vi "AD（V2.0）.vi"() -> (1 "时域谱":dbl[](graph), 2 "幅频谱":dbl[](graph))   [LabVIEW 2016]
uses:
  <vilib>/Analysis/2dsp.llb/Real FFT.vi
  <vilib>/Analysis/NI_AALPro.lvlib
panel:
  out "数值":i32
  # "[220，2000]"
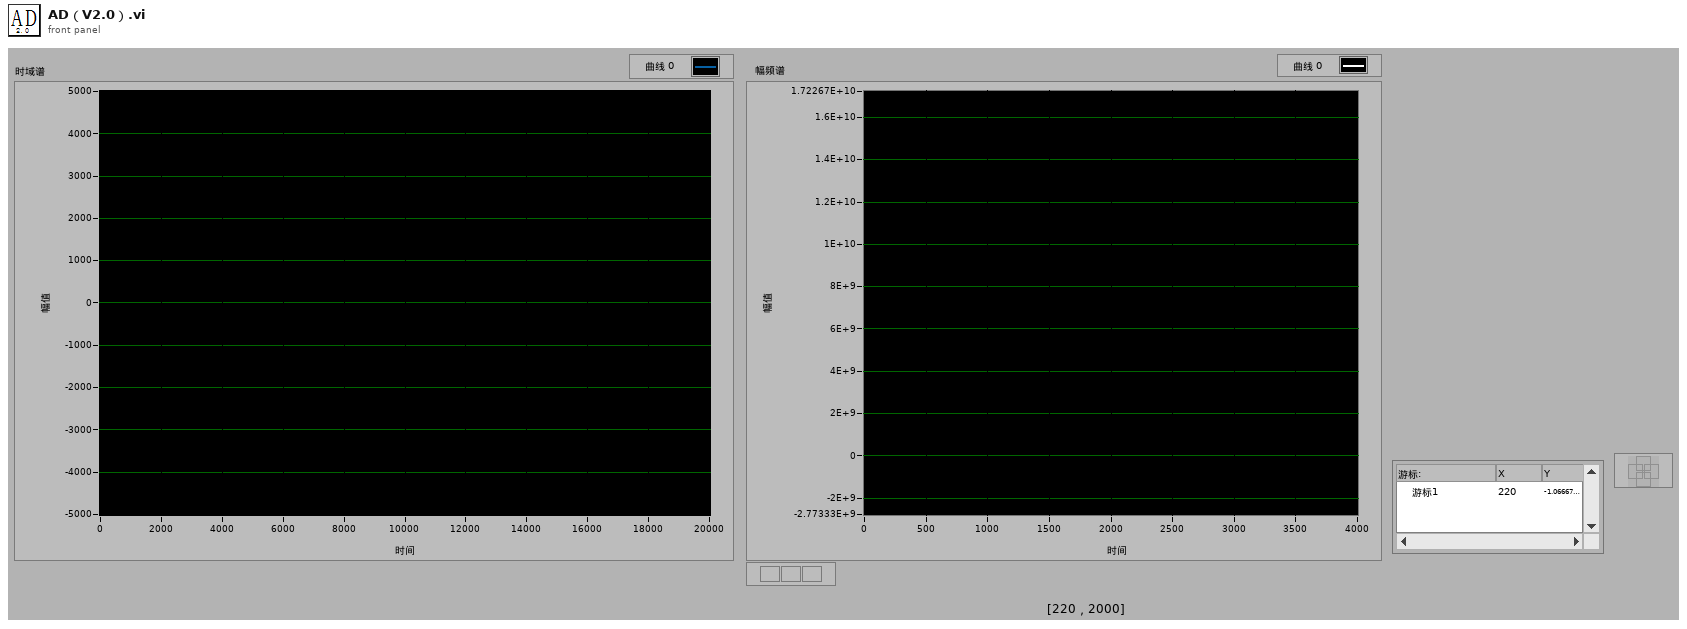
[diagram p1: front panel]
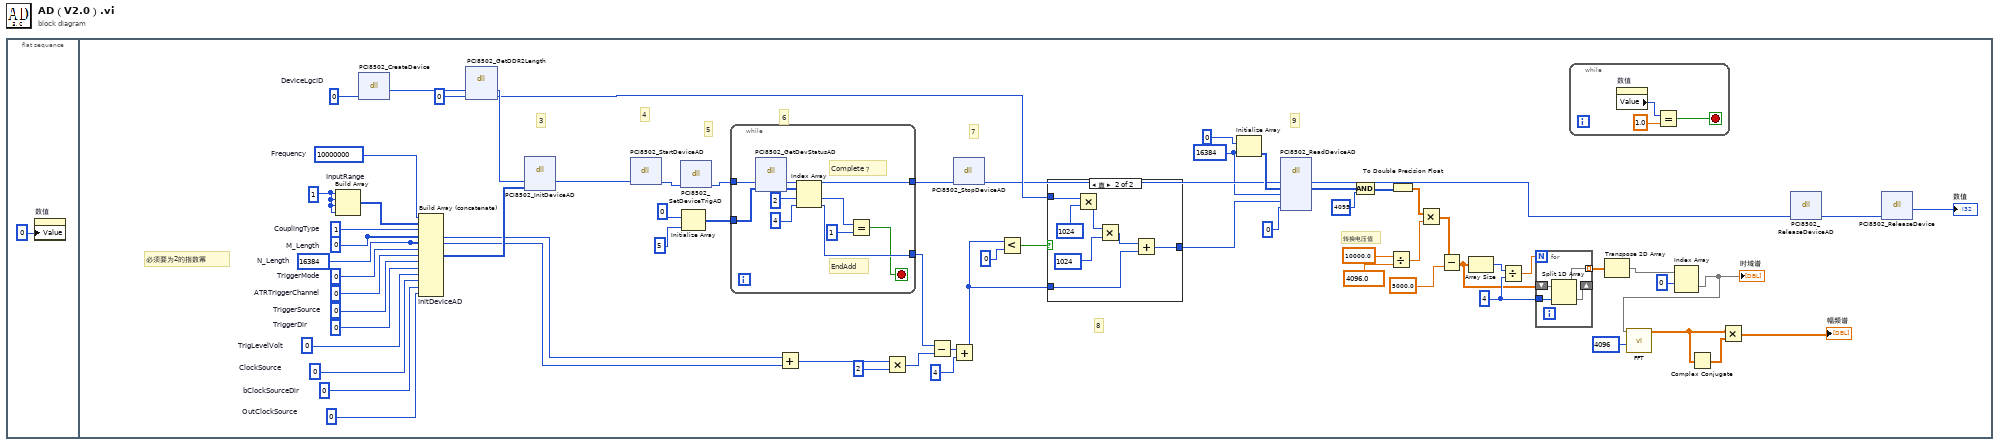
[diagram p0: block diagram]
diagram:
  n1 = flat-sequence {
    frame #0 {
      n2 = property on="数值" class="DigNum (严格)"("Value"=0 ("数值")) -> ()  [unwired: 2 in, 2 out]
    }
    frame #1 {
      w2 = 0  # DeviceLgcID
      w16 = 4
      w18 = 16384 ("dimension size")
      w57 = 0  # OutClockSource
      w58 = 0  # bClockSourceDir
      w60 = 10000000  # Frequency
      w61 = 0  # ClockSource
      w62 = 0  # TrigLevelVolt
      w5 = 1
      w63 = 0  # TriggerDir
      w64 = 0  # TriggerSource
      w65 = 0  # ATRTriggerChannel
      w66 = 0  # TriggerMode
      w49 = 16384  # N_Length
      w50 = 0  # M_Length
      w67 = 1  # CouplingType
      # "9"
      # "8"
      # "7"
      # "6"
      # "5"
      # "4"
      # "转换电压值"
      # "3"
      # "必须要为2的指数幂"
      n3 = Build Array "InputRange"(w5, w5, w5, w5) -> (w4:i32[])
      n4 = dll-call lib="PTH2]abs CUsersH301Desktopart闭环扫描程序采集卡控制INFamd64\nPCI8502_32" fn="PCI8502_CreateDevice" label="CreateDevice"("DeviceLgcID"=w2) -> (w55:i32)  [unwired: 4 in, 2 out]
      n5 = Build Array (concatenate) "InitDeviceAD"(w60, w4, w67, w50, w49, w66, w65, w64, w63, w62, w61, w58, w57) -> (w59:i32[])
      n6 = dll-call lib="PTH2]abs CUsersH301Desktopart闭环扫描程序采集卡控制INFamd64\nPCI8502_32" fn="PCI8502_GetDDR2Length" label="GetDDR2Length"("hDevice"=w55, "pulDDR2Length"=u32 0) -> ("hDevice"=w54:i32, "pulDDR2Length"=w52:u32)  [unwired: 4 in, 2 out]
      n7 = dll-call lib="PTH2]abs CUsersH301Desktopart闭环扫描程序采集卡控制INFamd64\nPCI8502_32" fn="PCI8502_InitDeviceAD" label="InitDeviceAD"("hDevice"=w54, "pADPara"=w59) -> ("hDevice"=w56:i32)  [unwired: 5 in, 2 out]
      n8 = dll-call lib="PTH2]abs CUsersH301Desktopart闭环扫描程序采集卡控制INFamd64\nPCI8502_32" fn="PCI8502_StartDeviceAD" label="StartDeviceAD"("hDevice"=w56) -> ("hDevice"=w47:i32)  [unwired: 4 in, 2 out]
      n9 = dll-call lib="PTH2]abs CUsersH301Desktopart闭环扫描程序采集卡控制INFamd64\nPCI8502_32" fn="PCI8502_SetDeviceTrigAD" label="SetDeviceTrigAD"("hDevice"=w47) -> ("hDevice"=w25:i32)  [unwired: 4 in, 2 out]
      n10 = Initialize Array(0, 5) -> (w22:i32[])
      n11 = while {
        tunnel: [w79] -> w21
        tunnel: w25 -> [w78]
        tunnel: w22 -> [w77]
        tunnel: [w76] -> w19
        stop <- w75 stop-if-true
        # "EndAdd"
        # "Complete？"
        n12 = dll-call lib="PTH2]abs CUsersH301Desktopart闭环扫描程序采集卡控制INFamd64\nPCI8502_32" fn="PCI8502_GetDevStatusAD" label="GetDevStatusAD"("hDevice"=w78, "pADStatus"=w77) -> ("hDevice"=w76:i32, "pADStatus"=w81:i32[])  [unwired: 4 in, 2 out]
        n13 = Index Array(array=w81, index #1=2, index #2=4) -> (element #1=w83:i32, element #2=w79:i32)
        n14 = Equal?(x=w83, y=1) -> (x = y?=w75:bool)
      }
      n15 = Add(x=w50, y=w49) -> (x+y=w20:i32)
      n16 = Multiply(x=w20, y=u32 2) -> (x*y=w33:u32)
      n17 = Subtract(x=w21, y=w33) -> (x-y=w35:u32)
      n18 = Add(x=w35, y=u32 4) -> (x+y=w30:u32)
      n19 = dll-call lib="PTH2]abs CUsersH301Desktopart闭环扫描程序采集卡控制INFamd64\nPCI8502_32" fn="PCI8502_StopDeviceAD" label="StopDeviceAD"("hDevice"=w19) -> ("hDevice"=w36:i32)  [unwired: 4 in, 2 out]
      n20 = Less?(x=w30, y=u32 0) -> (x < y?=w26:bool)
      n21 = case shown="真" w26 {
        tunnel: w30 -> [w85 w88]
        tunnel: [w85 w87] -> w31
        tunnel: w52 -> [_ w86]
        frame False {
        }
        frame True {
          n22 = Multiply(x=w86, y=u32 1024) -> (x*y=w91:u32)
          n23 = Multiply(x=w91, y=u32 1024) -> (x*y=w89:u32)
          n24 = Add(x=w89, y=w88) -> (x+y=w87:u32)
        }
      }
      n25 = Initialize Array(0, w18) -> (w37:i32[])
      n26 = dll-call lib="PTH2]abs CUsersH301Desktopart闭环扫描程序采集卡控制INFamd64\nPCI8502_32" fn="PCI8502_ReadDeviceAD" label="ReadDeviceAD"("hDevice"=w36, "ADBuffer"=w37, "nReadSizeWords"=w18, "ulStartAddr"=w31, "nRetSizeWords"=0) -> ("hDevice"=w48:i32, "ADBuffer"=w28:u16[])  [unwired: 7 in, 2 out]
      n27 = And(x=w28, y=4095) -> (x .and. y?=w39:i32[])
      n28 = Divide(x=10000.0, y=4096.0) -> (x/y=w41:dbl)
      n29 = To Double Precision Float(number=w39) -> (double precision float=w42:dbl[])
      n30 = Multiply(x=w42, y=w41) -> (x*y=w40:dbl[])
      n31 = Subtract(x=w40, y=5000.0) -> (x-y=w14:dbl[])
      n32 = Array Size(array=w14) -> (size(s)=w17:i32)
      n33 = Divide(x=w17, y=w16) -> (x/y=w15:dbl)
      n34 = for {
        N: w15 -> [_]
        tunnel: w16 -> [w74]
        shift-right: [w72] -> _
        shift-left: w14 -> [w73]
        tunnel: [w71] -> w13 mode=indexing
        n35 = Split 1D Array(array=w73, index=w74) -> (first subarray=w71:dbl[], second subarray=w72:dbl[])
      }
      n36 = while {
        stop <- w70 stop-if-true
        n37 = property on="数值" class="DigNum (严格)"() -> ("Value"=w68:i32)  [unwired: 2 in, 2 out]
        n38 = Equal?(x=w68, y=1.0) -> (x = y?=w70:bool)
      }
      n39 = Transpose 2D Array(2D array=w13) -> (transposed array=w11:dbl[][])
      n40 = Index Array(array=w11, index (row)=0 ("索引 (行)")) -> (element=w9:dbl[])  [unwired: 1 in]
      "时域谱" <- w9
      n41 = call-poly <vilib>:"FFT.vi"("FFT size"=4096 ("m"), "X"=w9) -> ("FFT {X}"=w8:cdb[])  [unwired: 8 in, 1 out]
      n42 = Complex Conjugate(1:w8) -> (0:w7:cdb[])
      n43 = Multiply(x=w8, y=w7) -> (x*y=→"幅频谱":cdb[])
      n44 = dll-call lib="PTH2]abs CUsersH301Desktopart闭环扫描程序采集卡控制INFamd64\nPCI8502_32" fn="PCI8502_ReleaseDeviceAD" label="ReleaseDeviceAD"("hDevice"=w48) -> ("hDevice"=w51:i32)  [unwired: 4 in, 2 out]
      n45 = dll-call lib="PTH2]abs CUsersH301Desktopart闭环扫描程序采集卡控制INFamd64\nPCI8502_32" fn="PCI8502_ReleaseDevice" label="ReleaseDevice"("hDevice"=w51) -> (→"数值":i32)  [unwired: 4 in, 2 out]
    }
  }
